vi "SVX Buffer Waterfall Graph.vi"   [LabVIEW 2017, in "SoundVib_SpectralDisplay.lvlib"]
doc: "Buffers signals and returns the buffered signals up to a maximum count. If you use this VI with the Waterfall Graph, the display mimics the behavior of a chart. Wire data to the <B>waterfall graph data</B> input to determine the polymorphic instance to use or manually select the instance."
uses:
  <vilib>/addons/Sound and Vibration/Order Analysis/Data Presentation/SoundVib_SpectralDisplay.lvlib
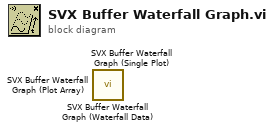
[diagram p0: block diagram]
diagram:
  n1 = call <vilib>:"SVX Buffer Waterfall Graph (Waterfall Data).vi"() -> ()  [unwired: 10 in, 2 out]
  n2 = call <vilib>:"SVX Buffer Waterfall Graph (Single Plot).vi"() -> ()  [unwired: 10 in, 2 out]
  n3 = call <vilib>:"SVX Buffer Waterfall Graph (Plot Array).vi"() -> ()  [unwired: 10 in, 2 out]
